vi "BitwiseNOTGreyscale.vi"(8 "error in (no error)":errorcluster, 9 "Mask":refnum<data-value>, 10 "Greyscale Image Destination":refnum<data-value>, 11 "Greyscale Image Source":refnum<data-value>) -> (0 "error out":errorcluster, 3 "Greyscale Image Destination (duplicate)":refnum<data-value>)   [LabVIEW 2020, in "g_ar_toolkit.image.lvlib"]
uses:
  g_ar_toolkit.image.lvlib
  f9ee80d6-438b-4cfb-91f1-04b98ac80474.vi
  <vilib>/Utility/error.llb/Error Cluster From Error Code.vi
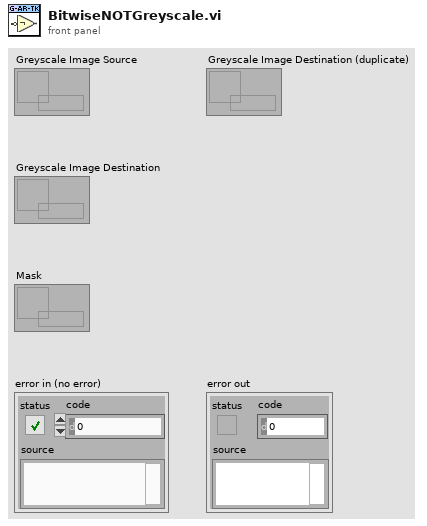
[diagram p1: front panel]
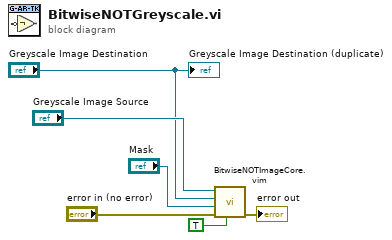
[diagram p0: block diagram]
diagram:
  n1 = call "BitwiseNOTImageCore.vim"("HasMask"=TRUE, "error in (no error)"="error in (no error)", "Mask"="Mask", "Greyscale Image Destination"="Greyscale Image Destination", "Greyscale Image Source"="Greyscale Image Source") -> ("error out"=→"error out":errorcluster)  [unwired: 6 in]
  "Greyscale Image Destination (duplicate)" <- "Greyscale Image Destination"
